vi "LP core 3ch.vi"(8 "reset":bool, 9 "coeff":i32, 10 "index":i16, 11 "data in":fxp<+/-,16,1>) -> (1 "output valid!":bool, 3 "data out":fxp<+/-,16,1>)   [LabVIEW 2018, in "SCTL.lvlib"]
uses:
  SCTL.lvlib
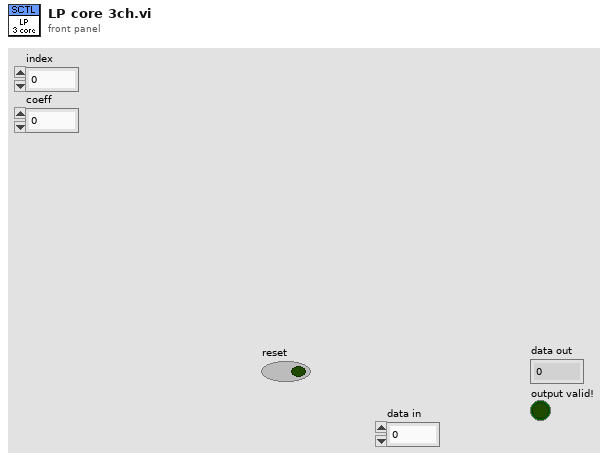
[diagram p1: front panel]
types:
  T1 = cluster{"A*B+C":i32, i32, "t":cluster{"y(n-2)":i32, "y/x2(n-1)":i32, "x(n-1)":i16, "x(n-2)":i16, "y2(n-1)":i32, "y2(n-2)":i32, "x2(n-2)":i32}}
  T2 = cluster{"y(n-2)":i32, "y/x2(n-1)":i32, "x(n-1)":i16, "x(n-2)":i16, "y2(n-1)":i32, "y2(n-2)":i32, "x2(n-2)":i32}
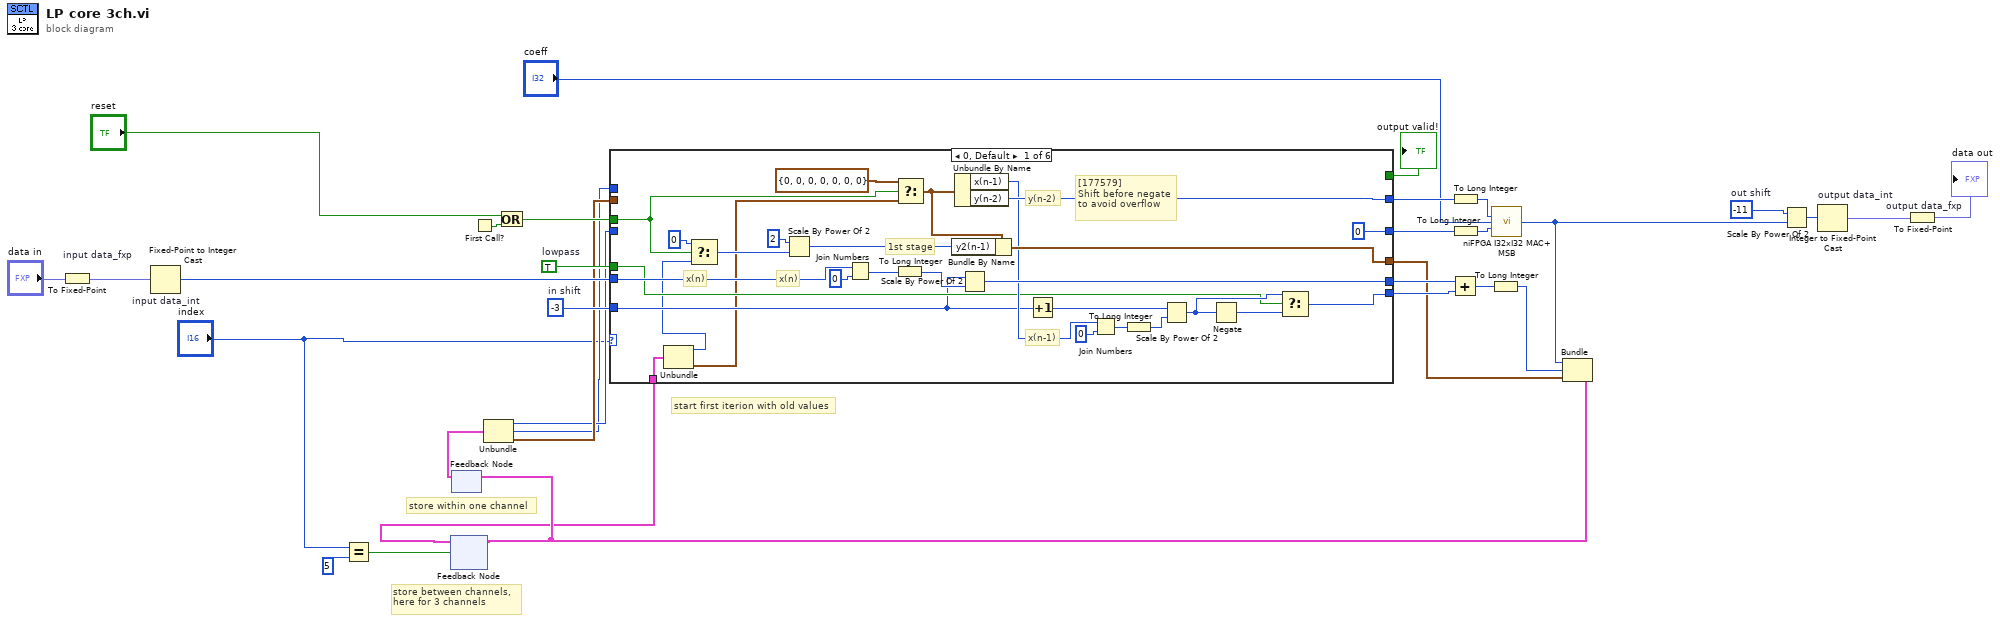
[diagram p0: block diagram]
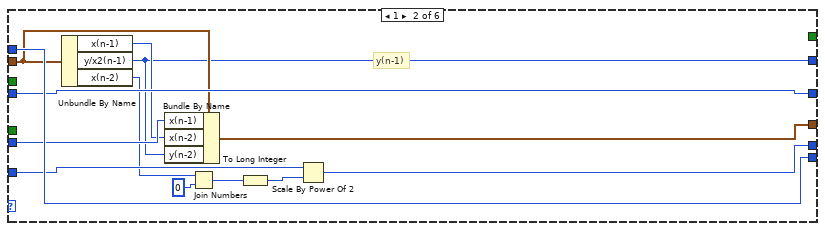
[diagram p2: hidden frame]
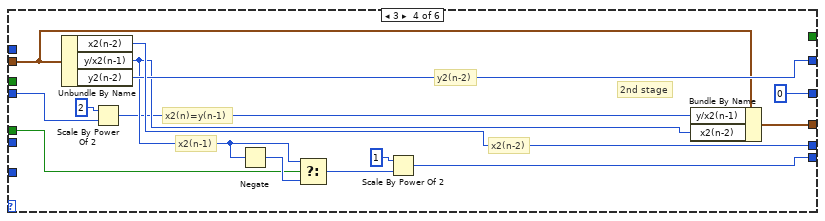
[diagram p4: hidden frame]
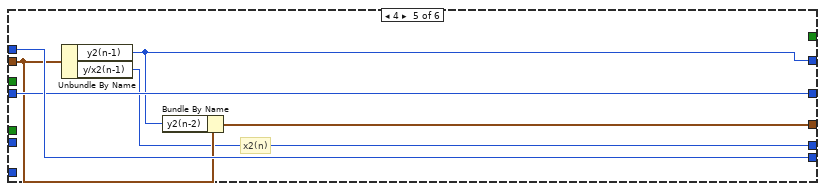
[diagram p5: hidden frame]
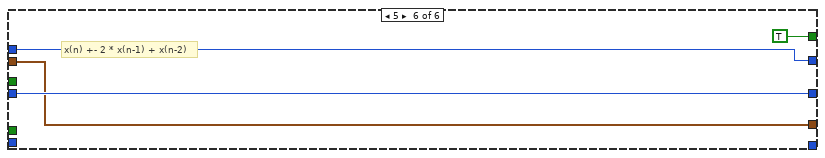
[diagram p6: hidden frame]
diagram:
  w19 = TRUE  # lowpass
  w21 = i8 -3  # in shift
  w27 = -11  # out shift
  # "start first iterion with old values"
  # "store between channels, \nhere for 3 channels"
  # "store within one channel"
  n1 = To Fixed-Point "input data_fxp"(number="data in") -> (fixed-point=w31:fxp<+/-,16,1>)  [unwired: 1 out]
  n2 = Fixed-Point to Integer Cast "input data_int"(1:w31) -> (0:w28:i16)
  n3 = Equal?(x="index", y=i16 5) -> (x = y?=w8:bool)
  n4 = feedback #1() -> (w2:T1)  [unwired: 1 in]
  n5 = feedback #2() -> (w1:T1)  [unwired: 1 in]
  n6 = First Call?() -> (First Call?: T/F=w20:bool)
  n7 = Unbundle(w1) -> ("A*B+C"=w5:i32, w4:i32, "t"=w6:T2)
  n8 = Or(x="reset", y=w20) -> (x .or. y?=w24:bool)
  n9 = case shown="0, Default" "index" {
    tunnel: [w61 w71 w75 w91 w93 w98] -> w10
    tunnel: w28 -> [w48 w70 _ _ _ _]
    tunnel: [w37 w74 _ w90 w97 _] -> w17
    tunnel: w4 -> [_ w74 w77 _ w97 w101]
    tunnel: [w58 w62 w77 w86 w95 w101] -> w15
    tunnel: [w47 w63 _ w88 w92 _] -> w18
    tunnel: [0 ("Numeric") w73 w76 0 ("Numeric") w96 w99] -> w16
    tunnel: [_ _ _ _ _ TRUE] -> w25
    tunnel: w24 -> [w52 _ _ _ _ _]
    tunnel: w5 -> [_ w73 w76 w80 w96 w99]
    tunnel: w6 -> [_ w72 w75 w81 w94 w98]
    tunnel: w21 -> [w40 w68 _ _ _ _]
    tunnel: w19 -> [w41 _ _ w83 _ _]
    tunnel: w2 -> [w36 _ _ _ _ _]
    frame 0, Default {
      # "[177579]\nShift before negate\nto avoid overflow"
      # "x(n)"
      # "1st stage"
      # "x(n)"
      # "x(n-1)"
      # "y(n-2)"
      n10 = Unbundle(w36) -> ("A*B+C"=w35:i32, "t"=w34:T2)  [unwired: 1 out]
      n11 = Select(t=0, s=w52, f=w35) -> (s? t:f=w53:i32)
      n12 = Scale By Power Of 2(n=2, x=w53) -> (x*2^n=w57:i32)
      n13 = Join Numbers(hi=w48, lo=i16 0) -> ((hi.lo)=w50:u32)
      n14 = To Long Integer(number=w50) -> (32bit integer=w49:i32)
      n15 = Select(t=T2 {"y(n-2)"=0, "y/x2(n-1)"=0, "x(n-1)"=0, "x(n-2)"=0, "y2(n-1)"=0, "y2(n-2)"=0, "x2(n-2)"=0}, s=w52, f=w34) -> (s? t:f=w55:T2)
      n16 = Bundle By Name(cluster=w55, "y2(n-1)"=w57) -> (w61:T2)
      n17 = Unbundle By Name(w55) -> ("x(n-1)"=w43:i16, "y(n-2)"=w58:i32)
      n18 = Scale By Power Of 2(n=w40, x=w49) -> (x*2^n=w47:i32)
      n19 = Increment(x=w40) -> (x+1=w39:i8)
      n20 = Join Numbers(hi=w43, lo=i16 0) -> ((hi.lo)=w44:u32)
      n21 = To Long Integer(number=w44) -> (32bit integer=w38:i32)
      n22 = Scale By Power Of 2(n=w39, x=w38) -> (x*2^n=w42:i32)
      n23 = Negate(x=w42) -> (-x=w46:i32)
      n24 = Select(t=w42, s=w41, f=w46) -> (s? t:f=w37:i32)
    }
    frame 1 {
      # "y(n-1)"
      n25 = Unbundle By Name(w72) -> ("x(n-1)"=w69:i16, "y/x2(n-1)"=w62:i32, "x(n-2)"=w66:i16)
      n26 = Bundle By Name(cluster=w72, "x(n-1)"=w70, "x(n-2)"=w69, "y(n-2)"=w62) -> (w71:T2)
      n27 = Join Numbers(hi=w66, lo=i16 0) -> ((hi.lo)=w65:u32)
      n28 = To Long Integer(number=w65) -> (32bit integer=w64:i32)
      n29 = Scale By Power Of 2(n=w68, x=w64) -> (x*2^n=w63:i32)
    }
    frame 2 {
      # "x(n) +- 2 * x(n-1) + x(n-2)"
    }
    frame 3 {
      # "2nd stage"
      # "x2(n)=y(n-1)"
      # "x2(n-2)"
      # "x2(n-1)"
      # "y2(n-2)"
      n30 = Unbundle By Name(w81) -> ("x2(n-2)"=w88:i32, "y/x2(n-1)"=w84:i32, "y2(n-2)"=w86:i32)
      n31 = Scale By Power Of 2(n=2, x=w80) -> (x*2^n=w79:i32)
      n32 = Negate(x=w84) -> (-x=w85:i32)
      n33 = Select(t=w84, s=w83, f=w85) -> (s? t:f=w82:i32)
      n34 = Scale By Power Of 2(n=1, x=w82) -> (x*2^n=w90:i32)
      n35 = Bundle By Name(cluster=w81, "y/x2(n-1)"=w79, "x2(n-2)"=w84) -> (w91:T2)
    }
    frame 4 {
      # "x2(n)"
      n36 = Unbundle By Name(w94) -> ("y2(n-1)"=w95:i32, "y/x2(n-1)"=w92:i32)
      n37 = Bundle By Name(cluster=w94, "y2(n-2)"=w95) -> (w93:T2)
    }
    frame 5 {
      # "x(n) +- 2 * x(n-1) + x(n-2)"
    }
  }
  "output valid!" <- w25
  n38 = Add(x=w18, y=w17) -> (x+y=w14:i32)
  n39 = To Long Integer(number=w15) -> (32bit integer=w22:i32)
  n40 = To Long Integer(number=w16) -> (32bit integer=w23:i32)
  n41 = To Long Integer(number=w14) -> (32bit integer=w11:i32)
  n42 = call <vilib>:"niFPGA I32xI32 MAC+ MSB.vi"("A"=w22, "B"="coeff", "C"=w23) -> ("A*B+C"=w12:i32)  [unwired: 12 in]
  n43 = Bundle("A*B+C"=w12, w11, "t"=w10) -> (w7:T1)  [unwired: 1 in]
  n44 = feedback-in #1(w7, w8) -> ()
  n45 = feedback-in #2(w7) -> ()
  n46 = Scale By Power Of 2(n=w27, x=w12) -> (x*2^n=w29:i32)
  n47 = Integer to Fixed-Point Cast "output data_int"(integer=w29) -> (fixed-point=w30:fxp<+/-,32,17>)  [unwired: 1 in]
  n48 = To Fixed-Point "output data_fxp"(number=w30) -> (fixed-point=→"data out":fxp<+/-,16,1>)  [unwired: 1 out]
